vi "DeleteTemporaryCryptedFolder.vi"(8 "error in (no error)":errorcluster, 11 "Folder_Mgmt":refnum<class "Folder_Mgmt.lvclass">) -> (0 "error out":errorcluster, 3 "Folder_Mgmt 2":refnum<class "Folder_Mgmt.lvclass">)   [LabVIEW 2016, in "Folder_Mgmt.lvclass"]
doc: "This VI deletes a DVR reference variable."
uses:
  Folder_Mgmt.lvclass
  C:/Users/Marco Preziani/Documents/DOME-LV16/Crypter/Crypter.lvclass
  Crypter/Crypter.lvclass/Crypter.ctl
  Crypter/Crypter.lvclass
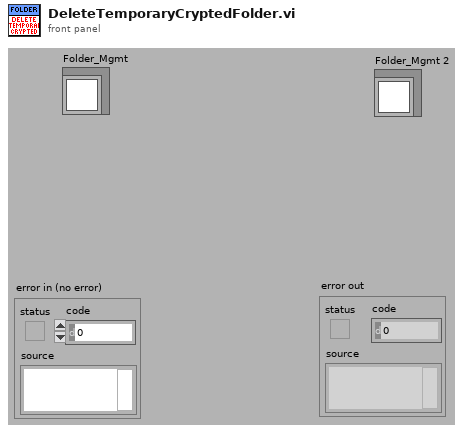
[diagram p1: front panel]
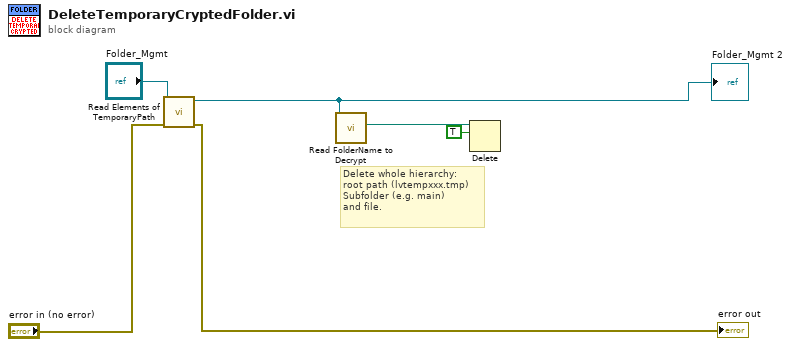
[diagram p0: block diagram]
diagram:
  # "Delete whole hierarchy:\nroot path (lvtempxxx.tmp)\nSubfolder (e.g. main)\nand file."
  n1 = call "Read Elements of TemporaryPath.vi"("error in (no error)"="error in (no error)", "Folder_Mgmt"="Folder_Mgmt") -> ("error out"=→"error out":errorcluster, "Folder_Mgmt 2"=w1:refnum<class "Folder_Mgmt.lvclass">)  [unwired: 7 in, 1 out]
  "Folder_Mgmt 2" <- w1
  n2 = call "Read FolderName to Decrypt.vi"("Crypter in"=w1) -> ("FolderName to Decrypt"=w2:path)  [unwired: 8 in, 2 out]
  n3 = Delete(path (use dialog)=w2, entire hierarchy (F)=TRUE) -> ()  [unwired: 3 in, 3 out]
